vi "LabVIEW Version to Path.vi"(8 "error in (no error)":errorcluster, 11 "Version":string) -> (0 "error out":errorcluster, 2 "Port":i32, 3 "Path":path)   [LabVIEW 2019, in "PostBuildSupport.lvclass"]
uses:
  PostBuildSupport.lvclass
  <vilib>/Utility/sysdir.llb/System Directory Type.ctl
  <vilib>/Utility/config.llb/Read Key (I32).vi
  <vilib>/Utility/config.llb/Read Key (String).vi
  <vilib>/Utility/config.llb/Read Key (Path).vi
  <vilib>/Utility/config.llb/NI_LVConfig.lvlib
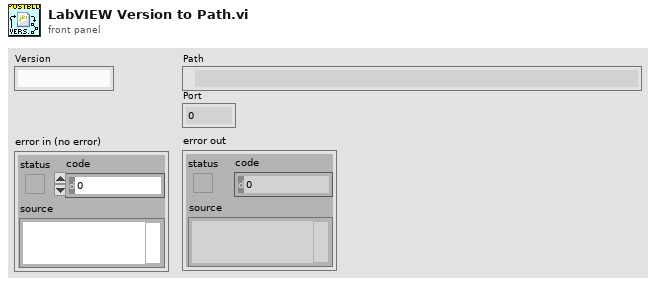
[diagram p1: front panel]
types:
  T1 = typedef "System Directory Type.ctl" = i32
  T2 = typedef "NI_LVConfig.lvlib/Config Data RefNum.ctl" = refnum<k1>
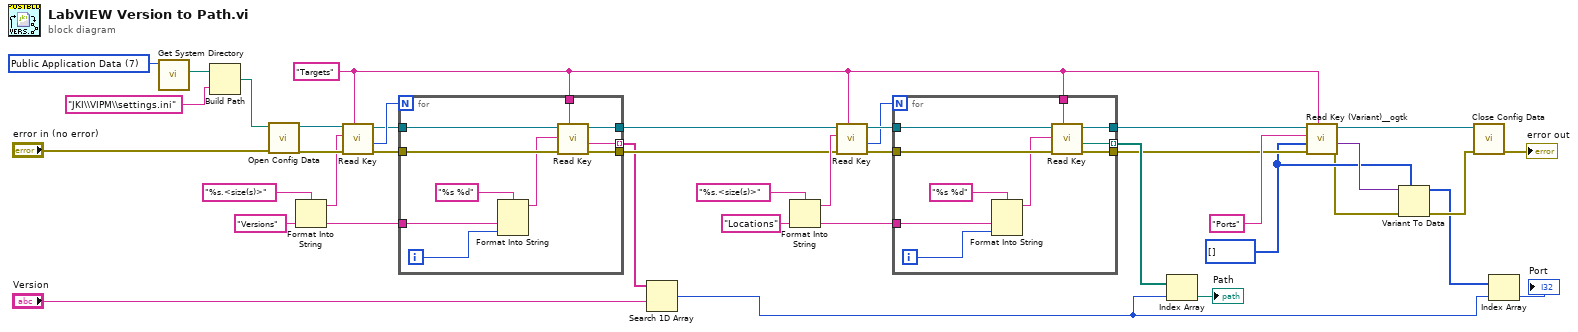
[diagram p0: block diagram]
diagram:
  w5 = i32[] [] ("index of element")
  w20 = "Locations" ("input 1")
  w28 = "Versions" ("input 1")
  w10 = "Targets" ("section")
  w38 = T1 7 items=["User Home"=0, "User Desktop"=1, "User Documents"=2, "User Application Data"=3, "User Preferences"=4, "User Temporary"=5, "Public Documents"=6, "Public Application Data"=7, "Public Preferences"=8, "Public Cache"=13, "System Core Libraries"=9, "System Installed Libraries"=10, "Application Files"=11, "Boot Volume Root"=12] ("system directory type")
  n1 = call <vilib>:"Get System Directory.vi"("system directory type"=w38) -> ("system directory"=w37:path)  [unwired: 10 in]
  n2 = Build Path(base path=w37, name or relative path="JKI\\VIPM\\settings.ini") -> (appended path=w14:path)
  n3 = call <vilib>:"Open Config Data.vi"("error in (no error)"="error in (no error)", "configuration file path"=w14) -> ("error out"=w34:errorcluster, "refnum"=w35:T2)  [unwired: 7 in, 1 out]
  n4 = Format Into String(format string="%s.<size(s)>", w28) -> (resulting string=w32:string)  [unwired: 2 in, 1 out]
  n5 = call-poly <vilib>:"Read Key.vi"("section"=w10, "error in (no error)"=w34, "key"=w32, "refnum"=w35) -> ("error out"=w29:errorcluster, "value"=w31:i32, "refnum out"=w30:T2)  [unwired: 4 in, 1 out]
  n6 = for {
    N: w31 -> [_]
    tunnel: w30 -> [w48]
    tunnel: w29 -> [w47]
    tunnel: w28 -> [w43]
    tunnel: w10 -> [w42]
    tunnel: [w41] -> w23
    tunnel: [w40] -> w22
    tunnel: [w39] -> w19 mode=indexing
    i -> [w44]
    n7 = Format Into String(format string="%s %d", w43, w44) -> (resulting string=w45:string)  [unwired: 2 in, 1 out]
    n8 = call-poly <vilib>:"Read Key.vi"("section"=w42, "error in (no error)"=w47, "key"=w45, "refnum"=w48) -> ("error out"=w40:errorcluster, "value"=w39:string, "refnum out"=w41:T2)  [unwired: 4 in, 1 out]
  }
  n9 = Search 1D Array(1D array=w19, element="Version") -> (index of element=w12:i32)  [unwired: 1 in]
  n10 = Format Into String(format string="%s.<size(s)>", w20) -> (resulting string=w24:string)  [unwired: 2 in, 1 out]
  n11 = call-poly <vilib>:"Read Key.vi"("section"=w10, "error in (no error)"=w22, "key"=w24, "refnum"=w23) -> ("error out"=w27:errorcluster, "value"=w25:i32, "refnum out"=w26:T2)  [unwired: 4 in, 1 out]
  n12 = for {
    N: w25 -> [_]
    tunnel: w26 -> [w58]
    tunnel: w27 -> [w57]
    tunnel: w20 -> [w53]
    tunnel: w10 -> [w52]
    tunnel: [w51] -> w17 mode=indexing
    tunnel: [w50] -> w8
    tunnel: [w49] -> w7
    i -> [w54]
    n13 = Format Into String(format string="%s %d", w53, w54) -> (resulting string=w55:string)  [unwired: 2 in, 1 out]
    n14 = call-poly <vilib>:"Read Key.vi"("section"=w52, "error in (no error)"=w57, "key"=w55, "refnum"=w58) -> ("error out"=w49:errorcluster, "value"=w51:path, "refnum out"=w50:T2)  [unwired: 4 in, 1 out]
  }
  n15 = Index Array(array=w17, index=w12) -> (element=→"Path":path)
  n16 = call <userlib>:"Read Key (Variant)__ogtk.vi"("section"=w10, "error in (no error)"=w7, "type"=w5, "key (optional)"="Ports" ("input 1"), "refnum"=w8) -> ("error out"=w4:errorcluster, "key-value"=w6:variant, "refnum out"=w9:T2)  [unwired: 3 in, 1 out]
  n17 = Variant To Data(error in=w4, type=w5, Variant=w6) -> (data=w2:i32[], error out=w3:errorcluster)
  n18 = call <vilib>:"Close Config Data.vi"("error in (no error)"=w3, "refnum"=w9) -> ("error out"=→"error out":errorcluster)  [unwired: 8 in, 1 out]
  n19 = Index Array(array=w2, index=w12) -> (element=→"Port":i32)
